vi "Splash Screen.vi"() -> ()   [LabVIEW 2017, in "TPP demo V2启动器.lvlib"]
uses:
  TPP demo V2/TPP demo V2/Load App.vi
  TPP demo V2/TPP demo V2/TPP demo V2.lvclass
panel:
  out "应用程序名称":string
  out "等待指示灯":T1
  out "当前操作":string caption="当前操作："
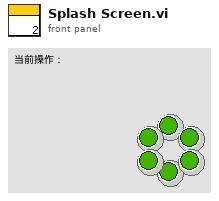
[diagram p1: front panel]
types:
  T1 = cluster{"等待1":bool, "等待2":bool, "等待3":bool, "等待4":bool, "等待5":bool, "等待6":bool}
  T2 = cluster{"[0]":bool, "[1]":bool, "[2]":bool, "[3]":bool, "[4]":bool, "[5]":bool}
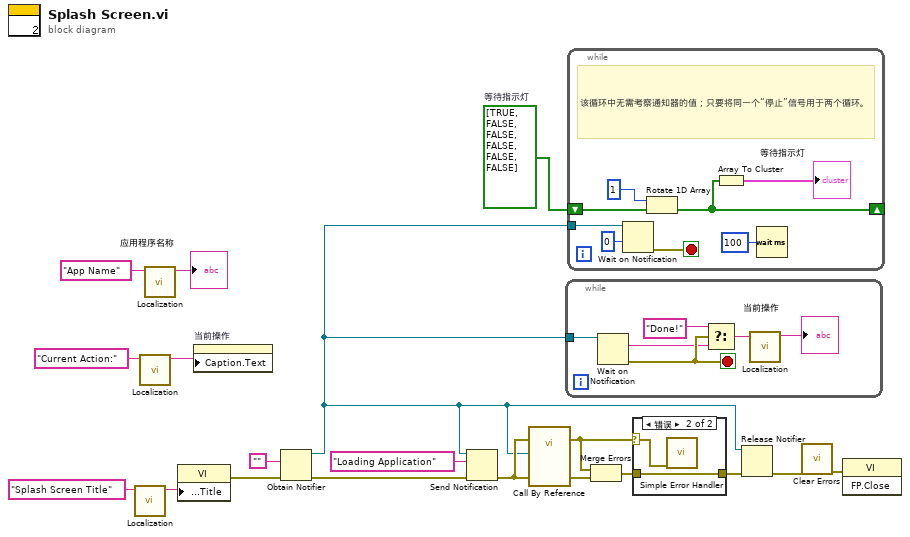
[diagram p0: block diagram]
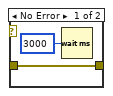
[diagram p2: hidden frame]
diagram:
  w12 = bool[] [TRUE, FALSE, FALSE, FALSE, FALSE, FALSE]  # 等待指示灯
  n1 = call "Localization.vi"("未本地化"="Splash Screen Title" ("Window Title")) -> ("本地化"=w19:string)  [unwired: 10 in]
  n2 = call "Localization.vi"("未本地化"="Current Action:" ("Window Title")) -> ("本地化"=w8:string)  [unwired: 10 in]
  n3 = call "Localization.vi"("未本地化"="App Name" ("Unlocalized")) -> ("本地化"=→"应用程序名称":string)  [unwired: 10 in]
  n4 = property class="VI"("Front Panel.Title"=w19) -> (error out=w17:errorcluster)  [unwired: 2 in, 1 out]
  n5 = property on="当前操作" class="Str"("Caption.Text"=w8) -> ()  [unwired: 2 in, 2 out]
  n6 = Obtain Notifier(notification data type="" ("Empty String Constant"), error in (no error)=w17) -> (notifier out=w2:refnum<notifier>, error out=w10:errorcluster)  [unwired: 2 in, 1 out]
  n7 = Send Notification(notification="Loading Application", notifier=w2, error in (no error)=w10) -> (error out=w5:errorcluster)  [unwired: 1 out]
  n8 = call-by-ref "?"(error in=w5, "错误输入（无错误）"=w5, "通知器"=w2) -> (error out=w4:errorcluster, 0:"error out"=w3:errorcluster)  [unwired: 10 in, 1 out]
  n9 = while {
    tunnel: w2 -> [w24]
    stop <- w23 stop-if-true
    n10 = Wait on Notification(notifier=w24) -> (notification=w21:string, error out=w23:errorcluster)  [unwired: 3 in, 2 out]
    n11 = Select(t="Done!" ("notification"), s=w23, f=w21) -> (s? t:f=w20:string)
    n12 = call "Localization.vi"("未本地化"=w20) -> ("本地化"=→"当前操作":string)  [unwired: 10 in]
  }
  n13 = while {
    shift-right: [w27] -> _
    shift-left: w12 -> [w29]
    tunnel: w2 -> [w31]
    stop <- w33 stop-if-true
    # "该循环中无需考察通知器的值；只要将同一个“停止”信号用于两个循环。"
    n14 = Wait on Notification(notifier=w31, timeout in ms (-1)=0) -> (error out=w33:errorcluster)  [unwired: 2 in, 3 out]
    n15 = Rotate 1D Array(1:w29, 2:1 ("n")) -> (0:w27:bool[])
    n16 = Array To Cluster(array=w27) -> (cluster=→"等待指示灯":T2)
    n17 = Wait (ms)(milliseconds to wait=u32 100) -> ()  [unwired: 1 out]
  }
  n18 = Merge Errors(w4, w3) -> (w6:errorcluster)
  n19 = case shown="错误" w4 {
    tunnel: [w35 w36] -> w7
    tunnel: w6 -> [w35 w36]
    selector: w4 -> [_ w37]
    frame No Error {
      n20 = Wait (ms)(milliseconds to wait=u32 3000) -> ()  [unwired: 1 out]
    }
    frame Error {
      n21 = call <vilib>:"Simple Error Handler.vi"("error in (no error)"=w37) -> ()  [unwired: 4 in, 5 out]
    }
  }
  n22 = Release Notifier(notifier=w2, error in (no error)=w7) -> (error out=w1:errorcluster)  [unwired: 1 in, 2 out]
  n23 = call <vilib>:"Clear Errors.vi"("error in (no error)"=w1) -> ("error out"=w11:errorcluster)  [unwired: 5 in, 1 out]
  n24 = invoke class="VI" method="FP.Close"(error in=w11) -> ()  [unwired: 2 in, 3 out]
